vi "K2602 Vsweep.vi"(6 "4-wire":bool, 8 "Settings":T1={"Channel"=enum."Channel A", "Vstart"=-2.0, "Vend"=0.5, "# of points"=30, "NPLC"=1.0, "I compliance"=0.001, "Delay ms"=500.0}, 11 "SMU":refnum<visa-resource-name>="GPIB0::26::INSTR") -> (0 "error out":errorcluster, 2 "V":dbl[](array[numeric])=[-2.0, -1.91379, -1.82759, -1.74138, -1.65517, -1.56897, -1.48276, -1.39655, -1.31034, -1.22414, -1.13793, -1.05172, -0.965517, -0.87931, -0.793103, -0.706896, -0.620689, -0.534482, -0.448276, -0.362069, -0.275862, -0.189655, -0.103448, -0.017241, 0.0689659, 0.155173, 0.24138, 0.327587, 0.413793, 0.5], 3 "I":dbl[](array[numeric])=[-0.000999973, -0.000999974, -0.000999972, -0.000999975, -0.000999974, -0.000999974, -0.000999972, -0.000999972, -0.000999971, -0.00099997, -0.000999971, -0.000999971, -0.000896573, -0.000729816, -0.000581092, -0.000448576, -0.00033406, -0.000237333, -0.000158658, -9.76653e-05, -5.40818e-05, -2.54308e-05, -9.0436e-06, -1.46604e-06, 5.28751e-06, 3.04662e-05, 0.000137424, 0.000464883, 0.000999977, 0.00099998])   [LabVIEW 2012]
uses:
  <instrlib>/KE26XX/KE26XX.lvlib
panel:
  out "Final Script":string="smu = smua\r\nsmusense = smu.SENSE_LOCAL\r\nstartv = -2.000000E+0\r\nstopv = 5.000000E-1\r\npoints = 30\r\nnplc = 1.000000E+0\r\nirange = 1.000000E-3\r\ndwell = 5.000000E-1\r\n-- Configure SMU\n smu.reset()\n smu.measure.nplc\t\t=nplc\n\tsmu.measure.autozero\t= smu.AUTOZERO_ONCE\n\tsmu.measure.autorangei\t= smu.AUTORANGE_ON\n\tsmu.source.autorangev\t= smu.AUTORANGE_ON\n smu.source.limiti = irange\n smu.sense = smusense\n\nfunction SweepVLinMeasureI(smu, startv, stopv, stime, points)\n    -- Default to smua if no smu is specified.\n    if smu == nil then\n        smu = smua\n    end\n\n    -- Save settings in temporary variables so they can be restored at the end.\n    local l_s_levelv = smu.source.levelv \n    local l_s_rangev = smu.source.rangev\n    local l_s_autorangev = smu.source.autorangev \n    local l_s_func = smu.source.func\n    local l_m_autozero = smu.measure.autozero\n    local l_d_screen = display.screen\n\n    -- Temporary variables used by this function.\n    local l_j, l_stepv, l_sweepv\n\n    -- Clear the front panel display then prompt for input parameters if missing.\n    display.clear()  \n    if startv == nil then\n        startv = display.prompt(l_volts_fmt, \" Volts\", \"Enter START voltage.\", -1, -l_max_volts, l_max_volts)\n        if startv == nil then\n            --Abort if Exit key pressed\n            AbortScript(l_d_screen)\n        end\n    end\n    if stopv == nil then\n        stopv = display.prompt(l_volts_fmt, \" Volts\", \"Enter STOP voltage.\", 1, -l_max_volts, l_max_volts)\n        if stopv == nil then\n            --Abort if Exit key pressed\n            AbortScript(l_d_screen)\n        end\n    end\n    if stime == nil then\n        stime = display.prompt(\"+0.000E+00\", \" Seconds\", \"Enter SETTLING time.\", 0, 0, 10)\n        if stime == nil then\n            --Abort if Exit key pressed\n            AbortScript(l_d_screen)\n        end\n    end\n    if points == nil then\n        points = display.prompt(\"0000\", \" Points\", \"Enter number of sweep POINTS.\", 10, 1, 1000)    \n        if points == nil then\n            --Abort if Exit key pressed\n            AbortScript(l_d_screen)\n        end\n    end\n    l_stepv = (stopv - startv)/(points - 1)\n    l_sweepv = startv   \n    \n    -- Update display with test info.\n    display.settext(\"Test Team Kicks Ass\")  -- Line 1 (20 characters max)\n    \n    -- Configure source and measure settings.\n    smu.source.output = smu.OUTPUT_OFF\n    smu.source.func = smu.OUTPUT_DCVOLTS\n    smu.source.levelv = 0\n    smu.source.rangev = math.max(math.abs(startv), math.abs(stopv))\n    smu.measure.autozero = smu.AUTOZERO_OFF\n    \n    -- Setup a buffer to store the result(s) in and start testing.\n    smu.nvbuffer1.clear()\n    smu.nvbuffer1.appendmode = 1\n    smu.nvbuffer1.collecttimestamps = 1\n    smu.nvbuffer1.collectsourcevalues = 1\n    smu.source.output = smu.OUTPUT_ON\n    for l_j = 1,points do\n        smu.source.levelv = l_sweepv  -- Program source to sweep level.\n        delay(stime)                  -- Wait desired settling time.\n        smu.measure.i(smu.nvbuffer1)  -- Measure current and store in reading buffer.\n        l_sweepv = l_sweepv + l_stepv   \n    end\n    smu.source.output = smu.OUTPUT_OFF\n\n    -- Update the front panel display and restore modified settings.\n    display.setcursor(2,1)             \n    display.settext(\"Test complete.\")     -- Line 2 (32 characters max)\n    smu.source.levelv = 0\n    smu.source.rangev = l_s_rangev\n    smu.source.autorangev = l_s_autorangev \n    smu.source.func = l_s_func\n    smu.source.levelv = l_s_levelv\n    smu.measure.autozero = l_m_autozero\n    --delay(2)\n    display.clear()\n    display.screen = l_d_screen\nend\n\n\tsmu.source.output\t\t= 1\nSweepVLinMeasureI(smu, startv, stopv, dwell, points)\n\tsmu.source.output\t\t= 0"
  in  "Sweep Script":string="-- Configure SMU\n smu.reset()\n smu.measure.nplc\t\t=nplc\n\tsmu.measure.autozero\t= smu.AUTOZERO_ONCE\n\tsmu.measure.autorangei\t= smu.AUTORANGE_ON\n\tsmu.source.autorangev\t= smu.AUTORANGE_ON\n smu.source.limiti = irange\n smu.sense = smusense\n\nfunction SweepVLinMeasureI(smu, startv, stopv, stime, points)\n    -- Default to smua if no smu is specified.\n    if smu == nil then\n        smu = smua\n    end\n\n    -- Save settings in temporary variables so they can be restored at the end.\n    local l_s_levelv = smu.source.levelv \n    local l_s_rangev = smu.source.rangev\n    local l_s_autorangev = smu.source.autorangev \n    local l_s_func = smu.source.func\n    local l_m_autozero = smu.measure.autozero\n    local l_d_screen = display.screen\n\n    -- Temporary variables used by this function.\n    local l_j, l_stepv, l_sweepv\n\n    -- Clear the front panel display then prompt for input parameters if missing.\n    display.clear()  \n    if startv == nil then\n        startv = display.prompt(l_volts_fmt, \" Volts\", \"Enter START voltage.\", -1, -l_max_volts, l_max_volts)\n        if startv == nil then\n            --Abort if Exit key pressed\n            AbortScript(l_d_screen)\n        end\n    end\n    if stopv == nil then\n        stopv = display.prompt(l_volts_fmt, \" Volts\", \"Enter STOP voltage.\", 1, -l_max_volts, l_max_volts)\n        if stopv == nil then\n            --Abort if Exit key pressed\n            AbortScript(l_d_screen)\n        end\n    end\n    if stime == nil then\n        stime = display.prompt(\"+0.000E+00\", \" Seconds\", \"Enter SETTLING time.\", 0, 0, 10)\n        if stime == nil then\n            --Abort if Exit key pressed\n            AbortScript(l_d_screen)\n        end\n    end\n    if points == nil then\n        points = display.prompt(\"0000\", \" Points\", \"Enter number of sweep POINTS.\", 10, 1, 1000)    \n        if points == nil then\n            --Abort if Exit key pressed\n            AbortScript(l_d_screen)\n        end\n    end\n    l_stepv = (stopv - startv)/(points - 1)\n    l_sweepv = startv   \n    \n    -- Update display with test info.\n    display.settext(\"Test Team Kicks Ass\")  -- Line 1 (20 characters max)\n    \n    -- Configure source and measure settings.\n    smu.source.output = smu.OUTPUT_OFF\n    smu.source.func = smu.OUTPUT_DCVOLTS\n    smu.source.levelv = 0\n    smu.source.rangev = math.max(math.abs(startv), math.abs(stopv))\n    smu.measure.autozero = smu.AUTOZERO_OFF\n    \n    -- Setup a buffer to store the result(s) in and start testing.\n    smu.nvbuffer1.clear()\n    smu.nvbuffer1.appendmode = 1\n    smu.nvbuffer1.collecttimestamps = 1\n    smu.nvbuffer1.collectsourcevalues = 1\n    smu.source.output = smu.OUTPUT_ON\n    for l_j = 1,points do\n        smu.source.levelv = l_sweepv  -- Program source to sweep level.\n        delay(stime)                  -- Wait desired settling time.\n        smu.measure.i(smu.nvbuffer1)  -- Measure current and store in reading buffer.\n        l_sweepv = l_sweepv + l_stepv   \n    end\n    smu.source.output = smu.OUTPUT_OFF\n\n    -- Update the front panel display and restore modified settings.\n    display.setcursor(2,1)             \n    display.settext(\"Test complete.\")     -- Line 2 (32 characters max)\n    smu.source.levelv = 0\n    smu.source.rangev = l_s_rangev\n    smu.source.autorangev = l_s_autorangev \n    smu.source.func = l_s_func\n    smu.source.levelv = l_s_levelv\n    smu.measure.autozero = l_m_autozero\n    --delay(2)\n    display.clear()\n    display.screen = l_d_screen\nend\n\n\tsmu.source.output\t\t= 1\nSweepVLinMeasureI(smu, startv, stopv, dwell, points)\n\tsmu.source.output\t\t= 0"
  in  "Read Points":u32=50
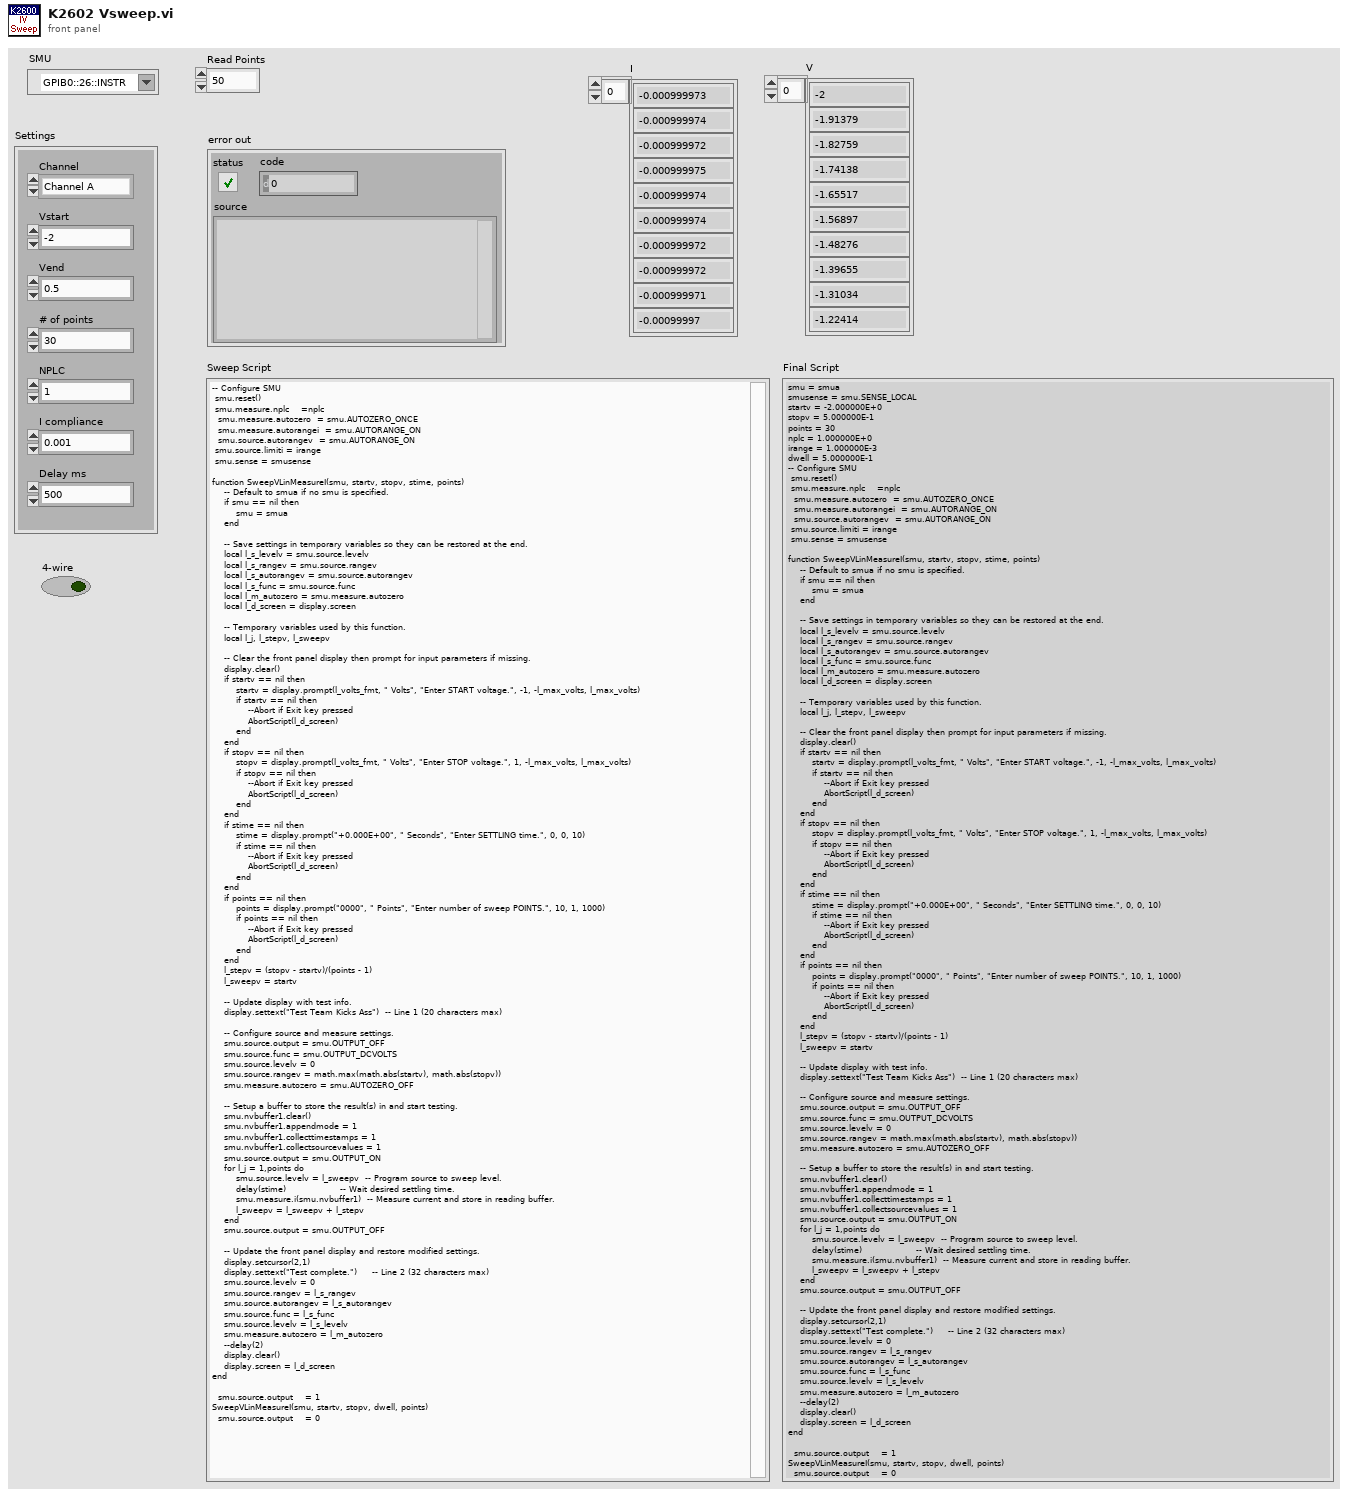
[diagram p1: front panel]
types:
  T1 = cluster{"Channel":enum32{"Channel A", "Channel B"}, "Vstart":dbl, "Vend":dbl, "# of points":u16, "NPLC":dbl, "I compliance":dbl, "Delay ms":dbl}
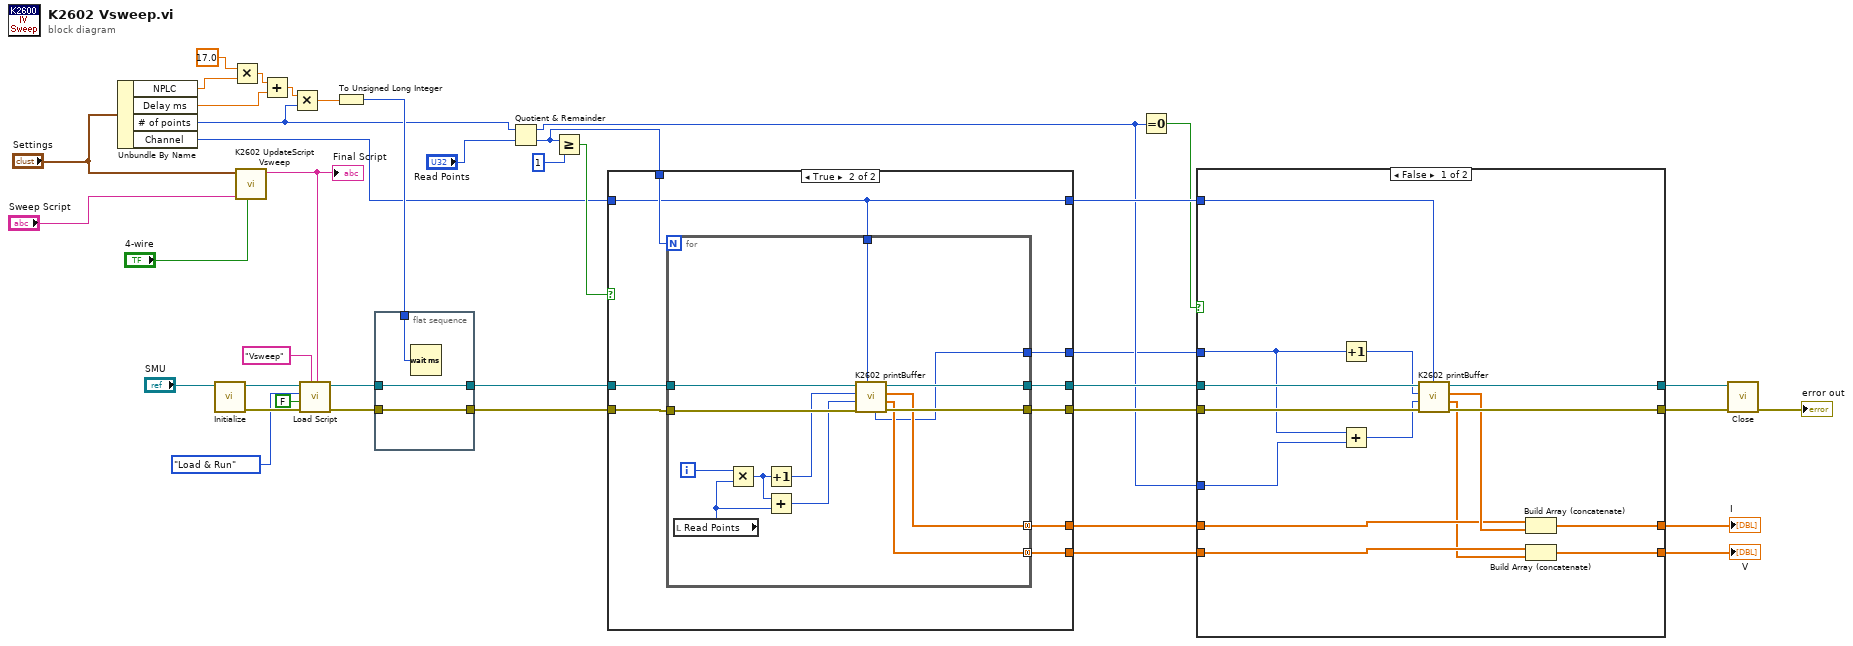
[diagram p0: block diagram]
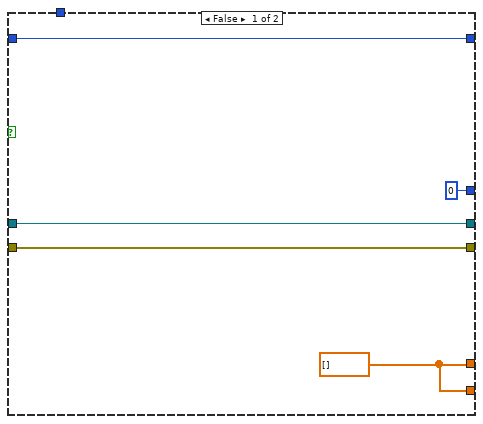
[diagram p3: hidden frame]
diagram:
  n1 = Unbundle By Name("Settings") -> ("NPLC"=w7:dbl, "Delay ms"=w5:dbl, "# of points"=w3:u16, "Channel"=w27:enum32{"Channel A", "Channel B"})
  n2 = call <instrlib>:"Initialize.vi"("VISA resource name"="SMU") -> ("error out"=w38:errorcluster, "VISA resource name out"=w39:refnum<visa-resource-name>)  [unwired: 9 in]
  n3 = Multiply(x=17.0, y=w7) -> (x*y=w6:dbl)
  n4 = call "K2602 UpdateScript Vsweep.vi"("4-wire"="4-wire", "Script"="Sweep Script", "Settings"="Settings") -> ("Output"=w8:string)  [unwired: 8 in]
  "Final Script" <- w8
  n5 = Add(x=w6, y=w5) -> (x+y=w4:dbl)
  n6 = Multiply(x=w4, y=w3) -> (x*y=w2:dbl)
  n7 = call <instrlib>:"Load Script.vi"("Script"=w8, "Script Name"="Vsweep", "error in"=w38, "Save (No)"=FALSE, "Load Options (Load)"=enum16{"Load", "Load & Run"}."Load & Run", "VISA resource name"=w39) -> ("error out"=w31:errorcluster, "VISA resource name out"=w32:refnum<visa-resource-name>)  [unwired: 4 out]
  n8 = To Unsigned Long Integer(number=w2) -> (unsigned 32bit integer=w33:u32)
  n9 = flat-sequence {
    tunnel: w33 -> [w43]
    tunnel: w32 -> [w42]
    tunnel: [w42] -> w25
    tunnel: w31 -> [w41]
    tunnel: [w41] -> w24
    frame #0 {
      n10 = Wait (ms)(milliseconds to wait=w43) -> ()  [unwired: 1 out]
    }
  }
  n11 = Quotient & Remainder(x=w3, y="Read Points") -> (x-y*floor(x/y)=w14:u32, floor(x/y)=w26:u32)
  n12 = Greater Or Equal?(x=w26, y=u32 1) -> (x >= y?=w28:bool)
  n13 = case shown="True" w28 {
    tunnel: w27 -> [w48 w52]
    tunnel: [w48 w52] -> w23
    tunnel: w26 -> [_ w57]
    tunnel: w25 -> [w47 w56]
    tunnel: w24 -> [w46 w55]
    tunnel: [w47 w54] -> w20
    tunnel: [w46 w53] -> w19
    tunnel: [w45 w51] -> w22
    tunnel: [w45 w50] -> w21
    tunnel: [u32 0 ("End Index out") w49] -> w12
    frame False {
      w45 = dbl[] [] ("array type (2D Dbl)")
    }
    frame True {
      n14 = for {
        N: w57 -> [_]
        tunnel: w56 -> [w70]
        tunnel: w55 -> [w69]
        tunnel: [w68] -> w54
        tunnel: [w67] -> w53
        tunnel: w52 -> [w66]
        tunnel: [w60] -> w51 mode=concatenating
        tunnel: [w59] -> w50 mode=concatenating
        tunnel: [w58] -> w49
        i -> [w65]
        n15 = local read "Read Points"() -> (w63:u32)
        n16 = Multiply(x=w65, y=w63) -> (x*y=w64:u32)
        n17 = Increment(x=w64) -> (x+1=w62:u32)
        n18 = Add(x=w64, y=w63) -> (x+y=w61:u32)
        n19 = call "K2602 printBuffer.vi"("Channel"=w66, "error in (no error)"=w69, "End Index"=w61, "Start Index"=w62, "SMU"=w70) -> ("error out"=w67:errorcluster, "V array"=w59:dbl[], "I array"=w60:dbl[], "SMU out"=w68:refnum<visa-resource-name>, "End Index out"=w58:u32)  [unwired: 2 in]
      }
    }
  }
  n20 = Equal To 0?(x=w14) -> (x = 0?=w13:bool)
  n21 = case shown="False" w13 {
    tunnel: w23 -> [w81 _]
    tunnel: w22 -> [w75 w87]
    tunnel: w21 -> [w73 w86]
    tunnel: w20 -> [w85 w89]
    tunnel: w19 -> [w84 w88]
    tunnel: [w83 w89] -> w18
    tunnel: [w82 w88] -> w17
    tunnel: [w74 w87] -> w11
    tunnel: [w71 w86] -> w16
    tunnel: w14 -> [w78 _]
    tunnel: w12 -> [w79 _]
    frame False {
      n22 = Increment(x=w79) -> (x+1=w80:u32)
      n23 = Add(x=w79, y=w78) -> (x+y=w77:u32)
      n24 = call "K2602 printBuffer.vi"("Channel"=w81, "error in (no error)"=w84, "End Index"=w77, "Start Index"=w80, "SMU"=w85) -> ("error out"=w82:errorcluster, "V array"=w72:dbl[], "I array"=w76:dbl[], "SMU out"=w83:refnum<visa-resource-name>)  [unwired: 2 in, 1 out]
      n25 = Build Array (concatenate)(w75, w76) -> (w74:dbl[])
      n26 = Build Array (concatenate)(w73, w72) -> (w71:dbl[])
    }
    frame True {
    }
  }
  "I" <- w11
  "V" <- w16
  n27 = call <instrlib>:"Close.vi"("error in (no error)"=w17, "VISA resource name"=w18) -> ("error out"=→"error out":errorcluster)  [unwired: 9 in]
